vi "list available jl functions.vi"(8 "error in (no error)":errorcluster) -> (0 "error out":errorcluster, 1 "Jl Server state out":T1, 3 "ext_fns":string[](array[string]), 4 "detailed error info":T2, 5 "return code":u8, 7 "timeout?":bool)   [LabVIEW 2018, in "LV-0mq-Julia_roundtrip-lib.lvlib" / "LV2Julia_core.lvlib"]
doc: "List function available on Server."
uses:
  LV2Julia_core.lvlib
  detailed error info.ctl
  StackFrame.ctl
  Server or client state.ctl
  318091ce-7b2e-4b52-a944-14c6363efdda.vi
  318091ce-7b2e-4b52-a944-14c6363efdda.vi/69b711a9-a39a-4729-98cc-e4df00af9649.vi
  318091ce-7b2e-4b52-a944-14c6363efdda.vi/69b711a9-a39a-4729-98cc-e4df00af9649.vi/f1fdd2dc-ce41-483a-9de5-fa9c36a5b59c.vi
  318091ce-7b2e-4b52-a944-14c6363efdda.vi/69b711a9-a39a-4729-98cc-e4df00af9649.vi/349bd2ca-23a5-40b6-8c9a-c29dc9b375f6.vi
  318091ce-7b2e-4b52-a944-14c6363efdda.vi/69b711a9-a39a-4729-98cc-e4df00af9649.vi/2b56d374-cd41-42bd-b243-a2bb3f16a3aa.vi
  check ID validity.vi
  bindata_descr to JSON.vi
  check cluster field names.vi
  concat JSON.vi
  build request.vi
  REQ full lifecycle.vi
  Parse server response.vi
  log jl exceptions.vi
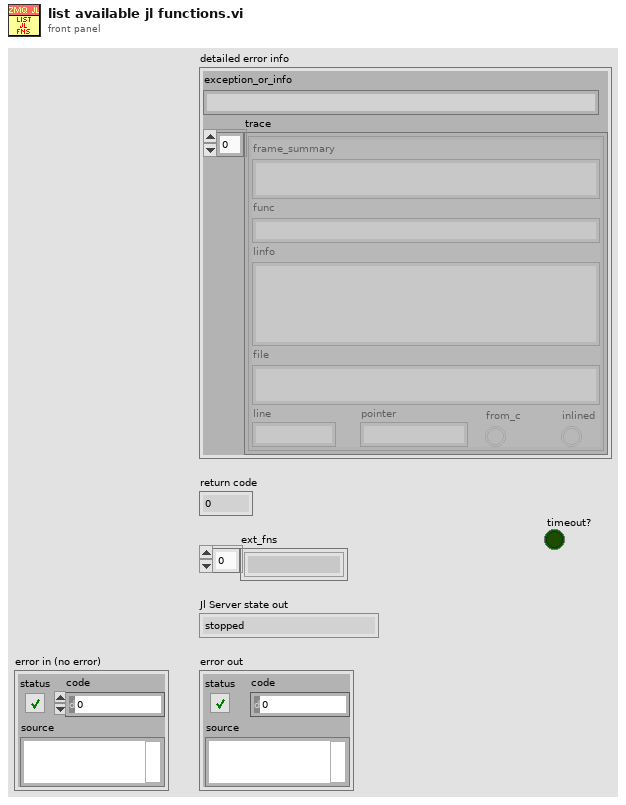
[diagram p1: front panel]
types:
  T1 = typedef "LV-0mq-Julia_roundtrip-lib.lvlib/LV2Julia_core.lvlib/Server or client state.ctl" = enum16{"stopped", "running", "unknown"}
  T2 = typedef "LV-0mq-Julia_roundtrip-lib.lvlib/LV2Julia_core.lvlib/detailed error info.ctl" = cluster{"exception_or_info":string, "trace":T3[]}
  T3 = typedef "LV-0mq-Julia_roundtrip-lib.lvlib/LV2Julia_core.lvlib/StackFrame.ctl" = cluster{"frame_summary":string, "func":string, "linfo":string, "file":string, "line":i32, "pointer":u64, "from_c":bool, "inlined":bool}
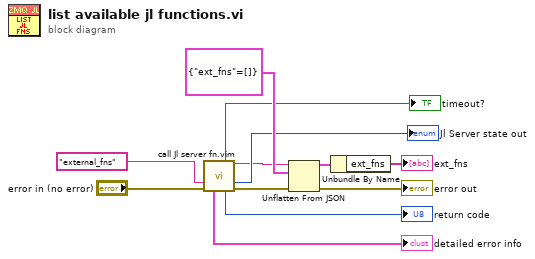
[diagram p0: block diagram]
diagram:
  n1 = call "call Jl server fn.vim"("fun2call"="external_fns", "error in (no error)"="error in (no error)") -> ("timeout?"=→"timeout?":bool, "JSON received"=w2:string, "Jl Server state out"=→"Jl Server state out":T1, "detailed error info"=→"detailed error info":T2, "return code"=→"return code":u8, "error out"=w3:errorcluster)  [unwired: 7 in, 1 out]
  n2 = Unflatten From JSON(JSON string=w2, type and defaults=cluster{"ext_fns":string[]} {"ext_fns"=[]}, error in (no error)=w3) -> (value=w11:cluster{"ext_fns":string[]}, error out=→"error out":errorcluster)  [unwired: 4 in]
  n3 = Unbundle By Name(w11) -> ("ext_fns"=→"ext_fns":string[])
